vi "Write Custom Char.vi"(8 "error in (no error)":errorcluster, 9 "Char":bool[][](array[boolean])=[[FALSE, FALSE, FALSE, FALSE, FALSE], [FALSE, FALSE, FALSE, FALSE, FALSE], [FALSE, FALSE, FALSE, FALSE, FALSE], [FALSE, FALSE, FALSE, FALSE, FALSE], [FALSE, FALSE, FALSE, FALSE, FALSE], [FALSE, FALSE, FALSE, FALSE, FALSE], [FALSE, FALSE, FALSE, FALSE, FALSE], [FALSE, FALSE, FALSE, FALSE, FALSE]], 11 "Character LCD in":refnum<class "LEDMatrix.lvclass">) -> (0 "error out":errorcluster, 3 "Character LCD out":refnum<class "LEDMatrix.lvclass">)   [LabVIEW 2020, in "CTI-Peripheral.lvlib" / "LEDMatrix.lvclass"]
uses:
  LEDMatrix.lvclass
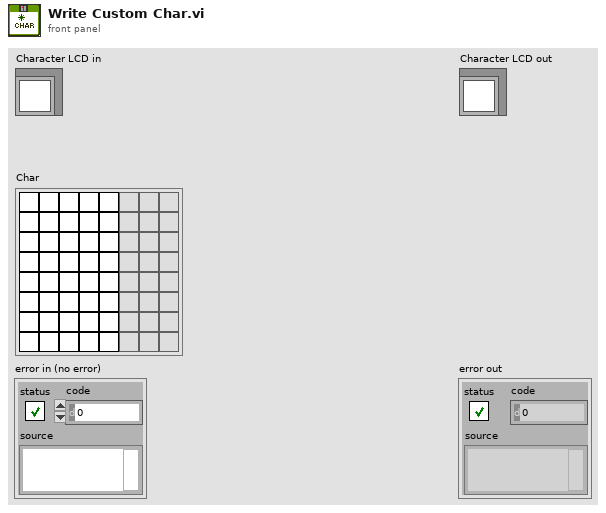
[diagram p1: front panel]
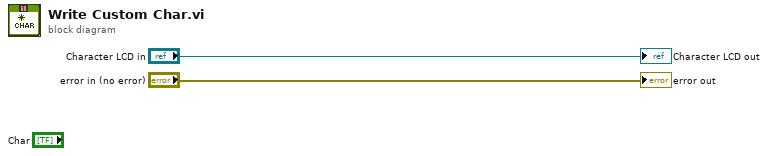
[diagram p0: block diagram]
diagram:
  "error out" <- "error in (no error)"
  "Character LCD out" <- "Character LCD in"
